vi "window_graph calc_intersect_point.vi"(2 "region data":cluster{"X":dbl, "Y":dbl}[](array[cluster]), 3 "limit data":cluster{"X":dbl, "Y":dbl}[](array[cluster])) -> (0 "vaild region data":cluster{"X":dbl, "Y":dbl}[](array[cluster]), 1 "baseline data":cluster{"X":dbl, "Y":dbl}[](array[cluster]))   [LabVIEW 2018]
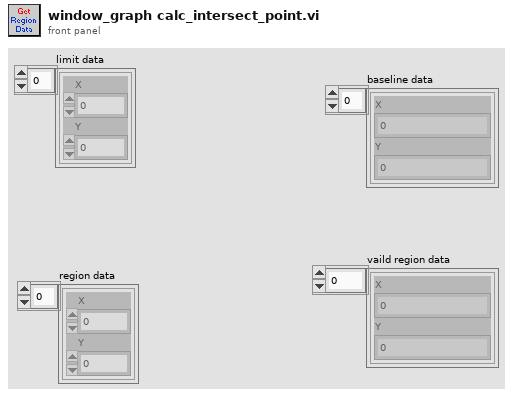
[diagram p1: front panel]
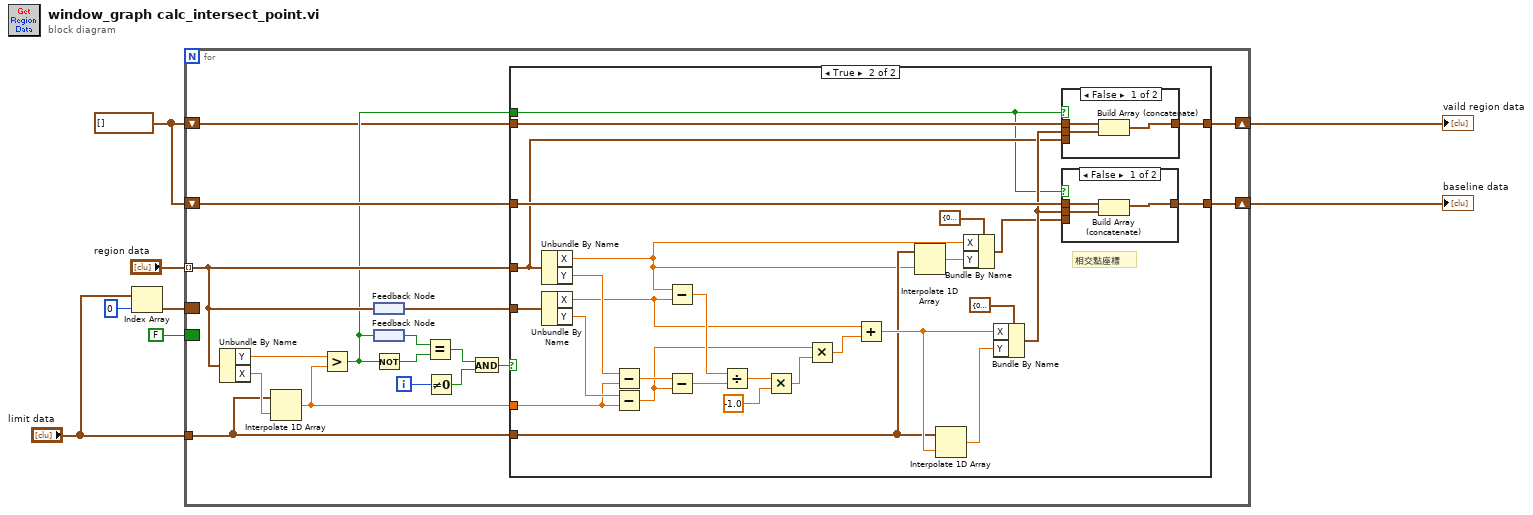
[diagram p0: block diagram]
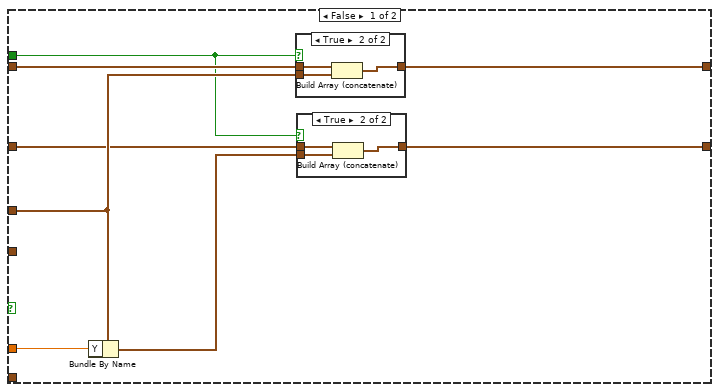
[diagram p2: hidden frame]
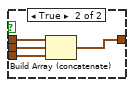
[diagram p5: hidden frame]
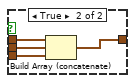
[diagram p6: hidden frame]
diagram:
  w4 = cluster{"X":dbl, "Y":dbl}[] []
  n1 = Index Array(array="limit data", index=0) -> (element=w6:cluster{"X":dbl, "Y":dbl})
  n2 = for {
    tunnel: "region data" -> [w19] mode=indexing
    tunnel: "limit data" -> [w18]
    border: w6 -> [_]
    border: FALSE -> [_]
    shift-right: [w16] -> w2
    shift-left: w4 -> [w13]
    shift-right: [w15] -> w1
    shift-left: w4 -> [w17]
    i -> [w12]
    n3 = Unbundle By Name(w19) -> ("Y"=w24:dbl, "X"=w25:dbl)
    n4 = Interpolate 1D Array(1:w25, 2:w18) -> (0:w21:dbl)
    n5 = Greater?(x=w24, y=w21) -> (0:w14:bool)
    n6 = feedback #1() -> (w20:cluster{"X":dbl, "Y":dbl})
    n7 = feedback-in #1(w19) -> ()
    n8 = feedback #2() -> (w23:bool)
    n9 = feedback-in #2(w14) -> ()
    n10 = Not(x=w14) -> (.not. x?=w22:bool)
    n11 = Equal?(x=w23, y=w22) -> (x = y?=w11:bool)
    n12 = Not Equal To 0?(x=w12) -> (x != 0?=w10:bool)
    n13 = And(x=w11, y=w10) -> (x .and. y?=w9:bool)
    n14 = case shown="True" w9 {
      tunnel: w19 -> [w31 w51]
      tunnel: w20 -> [_ w69]
      tunnel: w21 -> [w30 w66]
      tunnel: w18 -> [_ w46]
      tunnel: w17 -> [w28 w56]
      tunnel: [w32 w55] -> w16
      tunnel: [w26 w54] -> w15
      tunnel: w14 -> [w29 w47]
      tunnel: w13 -> [w33 w52]
      frame False {
        n15 = Bundle By Name(cluster=w31, "Y"=w30) -> (w27:cluster{"X":dbl, "Y":dbl})
        n16 = case shown="True" w29 {
          tunnel: w33 -> [w38 w41]
          tunnel: w31 -> [_ w40]
          tunnel: [w38 w39] -> w32
          frame False {
          }
          frame True {
            n17 = Build Array (concatenate)(w41, w40) -> (w39:cluster{"X":dbl, "Y":dbl}[])
          }
        }
        n18 = case shown="True" w29 {
          tunnel: w28 -> [w34 w37]
          tunnel: w27 -> [_ w36]
          tunnel: [w34 w35] -> w26
          frame False {
          }
          frame True {
            n19 = Build Array (concatenate)(w37, w36) -> (w35:cluster{"X":dbl, "Y":dbl}[])
          }
        }
      }
      frame True {
        # "相交點座標"
        n20 = Unbundle By Name(w51) -> ("X"=w44:dbl, "Y"=w68:dbl)
        n21 = Unbundle By Name(w69) -> ("X"=w60:dbl, "Y"=w67:dbl)
        n22 = Subtract(x=w68, y=w66) -> (x-y=w65:dbl)
        n23 = Subtract(x=w67, y=w66) -> (x-y=w48:dbl)
        n24 = Subtract(x=w44, y=w60) -> (x-y=w63:dbl)
        n25 = Subtract(x=w65, y=w48) -> (x-y=w64:dbl)
        n26 = Divide(x=w63, y=w64) -> (x/y=w61:dbl)
        n27 = Multiply(x=w61, y=-1.0 ("x-y")) -> (x*y=w50:dbl)
        n28 = Multiply(x=w48, y=w50) -> (x*y=w49:dbl)
        n29 = Add(x=w60, y=w49) -> (x+y=w58:dbl)
        n30 = Interpolate 1D Array(1:w44, 2:w46) -> (0:w43:dbl)
        n31 = Interpolate 1D Array(1:w58, 2:w46) -> (0:w57:dbl)
        n32 = Bundle By Name(cluster=cluster{"X":dbl, "Y":dbl} {"X"=0.0, "Y"=0.0} ("Position"), "X"=w44, "Y"=w43) -> (w42:cluster{"X":dbl, "Y":dbl})
        n33 = Bundle By Name(cluster=cluster{"X":dbl, "Y":dbl} {"X"=0.0, "Y"=0.0} ("Position"), "X"=w58, "Y"=w57) -> (w53:cluster{"X":dbl, "Y":dbl})
        n34 = case shown="False" w47 {
          tunnel: w53 -> [w78 w83]
          tunnel: w51 -> [_ w82]
          tunnel: w52 -> [w79 w81]
          tunnel: [w77 w80] -> w55
          frame False {
            n35 = Build Array (concatenate)(w79, w78) -> (w77:cluster{"X":dbl, "Y":dbl}[])
          }
          frame True {
            n36 = Build Array (concatenate)(w81, w83, w82) -> (w80:cluster{"X":dbl, "Y":dbl}[])
          }
        }
        n37 = case shown="False" w47 {
          tunnel: w56 -> [w72 w76]
          tunnel: [w70 w75] -> w54
          tunnel: w53 -> [w71 w74]
          tunnel: w42 -> [_ w73]
          frame False {
            n38 = Build Array (concatenate)(w72, w71) -> (w70:cluster{"X":dbl, "Y":dbl}[])
          }
          frame True {
            n39 = Build Array (concatenate)(w76, w74, w73) -> (w75:cluster{"X":dbl, "Y":dbl}[])
          }
        }
      }
    }
  }
  "baseline data" <- w1
  "vaild region data" <- w2
